vi "7SegmentMod3.vi"() -> ()   [LabVIEW 2014]
doc: "\"Discrete LED demo.vi\" -- Demonstrate a discrete LED connected to a digital output.\n\nInstructions:\n\n-- Click the 'enable blinker' button to toggle between blinking mode\nand static mode.\n-- In static mode, click the 'digital level' button to set the state of the\ndigital output.\n-- The 'digital output state' LED indicator shows the state of the\ndigital output (on = high, off = low)."
uses:
  <vilib>/Utility/error.llb/Error Cluster From Error Code.vi
  <vilib>/myRIO/Common/Instrument Driver Framework/myRIO v1.0/DIO/vis/myRIO v1.0 Write DIO.vi
  <vilib>/myRIO/Instrument Drivers/Onboard IO/DIO/DIO.lvlib
panel:
  in  "Figure-8 Speed":dbl=18.0
  in  "Direction: Figure-8":bool
  in  "Direction: Chase":bool
  in  "Path":enum16{"Chase", "Figure-8"}(ring)
  in  "Chase":dbl=18.0
  out "error out":errorcluster
  in  "error in (no error)":errorcluster
  in  "[ESC]":bool
  # "7-Segment LED demo"
  # "counter-clockwise"
  # "counter-clockwise"
  # "clockwise"
  # "clockwise"
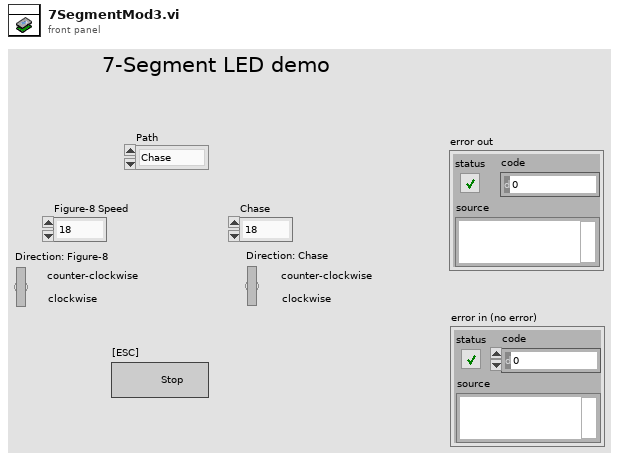
[diagram p1: front panel]
types:
  T1 = typedef "DIO.lvlib/DIO Reference.ctl" = cluster{"myRIO Reference":T2, "DIO Channels List":T6}
  T2 = typedef "myRIO Generic Hardware Reference.ctl" = cluster{"myRIO Model":T3, "myRIO Hardware Reference":T4}
  T3 = typedef "Hardware Version Enum.ctl" = enum16{"Unknown", "myRIO-1900", "myRIO-1950"}
  T4 = typedef "myRIO v1.0 Reference.ctl" = cluster{"Generic FPGA Reference":T5, "Allow multiple opens":bool}
  T5 = typedef "Generic FPGA Reference.ctl" = refnum<k20>
  T6 = typedef "DIO Channels List.ctl" = T7[]
  T7 = typedef "DIO Channels Enum.ctl" = enum16{"Not Connected", "C/DIO0", "C/DIO1", "C/DIO2", "C/DIO3", "C/DIO4", "C/DIO5", "C/DIO6", "C/DIO7", "A/DIO0", "A/DIO1", "A/DIO2", "A/DIO3", "A/DIO4", "A/DIO5", "A/DIO6", "A/DIO7", "A/DIO8", "A/DIO9", "A/DIO10", "A/DIO11", "A/DIO12", "A/DIO13", "A/DIO14", "A/DIO15", "B/DIO0", "B/DIO1", "B/DIO2", "B/DIO3", "B/DIO4", "B/DIO5", "B/DIO6", "B/DIO7", "B/DIO8", "B/DIO9", "B/DIO10", "B/DIO11", "B/DIO12", "B/DIO13", "B/DIO14", "B/DIO15", "LED0", "LED1", "LED2", "LED3", "Button0"}
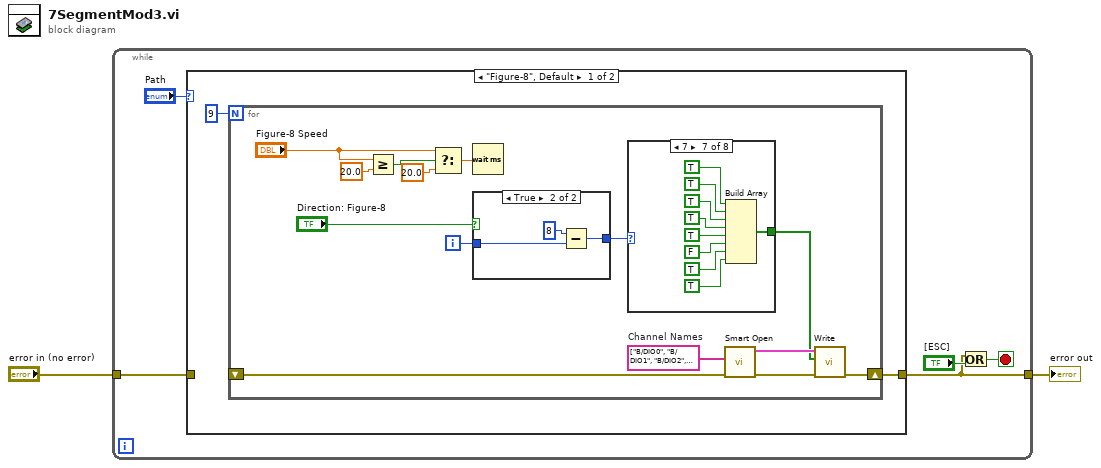
[diagram p0: block diagram]
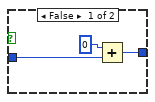
[diagram p2: hidden frame]
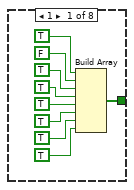
[diagram p3: hidden frame]
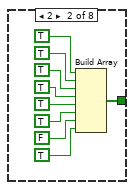
[diagram p4: hidden frame]
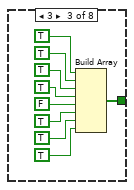
[diagram p5: hidden frame]
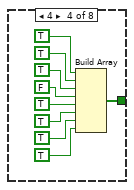
[diagram p6: hidden frame]
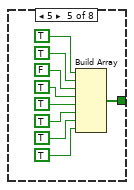
[diagram p7: hidden frame]
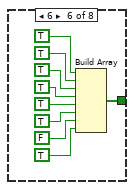
[diagram p8: hidden frame]
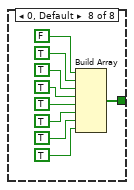
[diagram p9: hidden frame]
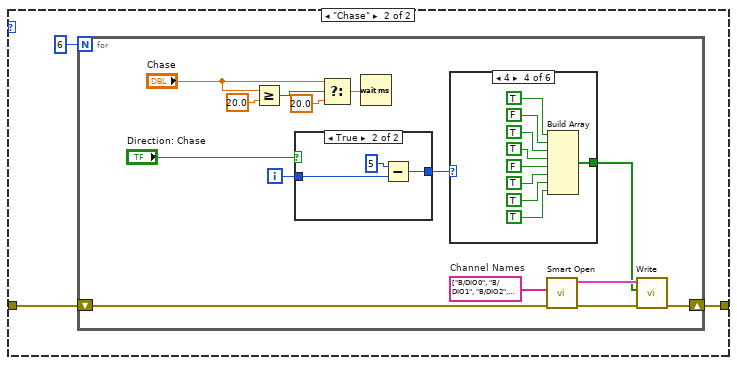
[diagram p10: hidden frame]
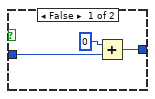
[diagram p11: hidden frame]
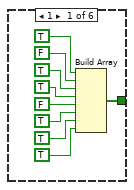
[diagram p12: hidden frame]
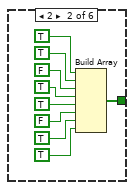
[diagram p13: hidden frame]
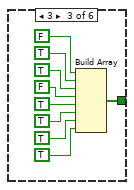
[diagram p14: hidden frame]
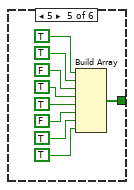
[diagram p15: hidden frame]
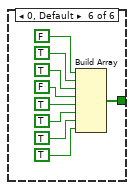
[diagram p16: hidden frame]
diagram:
  n1 = while {
    tunnel: [w5] -> w2
    tunnel: "error in (no error)" -> [w4]
    stop <- w7 stop-if-true
    n2 = case shown="\"Figure-8\", Default" "Path" {
      tunnel: [w8 w104] -> w5
      tunnel: w4 -> [_ w103]
      frame "Figure-8", Default {
        n3 = for {
          N: 9 -> [_]
          shift-right: [w22] -> w8
          shift-left: _ -> [w21]
          i -> [w12]
          w23 = tag[] ["B/DIO0", "B/DIO1", "B/DIO2", "B/DIO3", "B/DIO4", "B/DIO5", "B/DIO6", "B/DIO7"]  # Channel Names
          n4 = Greater Or Equal?(x="Figure-8 Speed", y=20.0) -> (x >= y?=w18:bool)
          n5 = Select(t="Figure-8 Speed", s=w18, f=20.0) -> (s? t:f=w16:dbl)
          n6 = Wait (ms)(milliseconds to wait=w16) -> ()  [unwired: 1 out]
          n7 = case shown="True" "Direction: Figure-8" {
            tunnel: [w25 w28] -> w11
            tunnel: w12 -> [w24 w27]
            frame False {
              n8 = Add(x=0, y=w24) -> (x+y=w25:i32)
            }
            frame True {
              n9 = Subtract(x=8, y=w27) -> (x-y=w28:i32)
            }
          }
          n10 = case shown="7" w11 {
            tunnel: [w30 w39 w48 w57 w66 w75 w84 w93] -> w13
            frame 1 {
              n11 = Build Array(TRUE, FALSE, TRUE, TRUE, TRUE, TRUE, TRUE, TRUE) -> (w30:bool[])
            }
            frame 2 {
              n12 = Build Array(TRUE, TRUE, TRUE, TRUE, TRUE, TRUE, FALSE, TRUE) -> (w39:bool[])
            }
            frame 3 {
              n13 = Build Array(TRUE, TRUE, TRUE, TRUE, FALSE, TRUE, TRUE, TRUE) -> (w48:bool[])
            }
            frame 4 {
              n14 = Build Array(TRUE, TRUE, TRUE, FALSE, TRUE, TRUE, TRUE, TRUE) -> (w57:bool[])
            }
            frame 5 {
              n15 = Build Array(TRUE, TRUE, FALSE, TRUE, TRUE, TRUE, TRUE, TRUE) -> (w66:bool[])
            }
            frame 6 {
              n16 = Build Array(TRUE, TRUE, TRUE, TRUE, TRUE, TRUE, FALSE, TRUE) -> (w75:bool[])
            }
            frame 7 {
              n17 = Build Array(TRUE, TRUE, TRUE, TRUE, TRUE, FALSE, TRUE, TRUE) -> (w84:bool[])
            }
            frame 0, Default {
              n18 = Build Array(FALSE, TRUE, TRUE, TRUE, TRUE, TRUE, TRUE, TRUE) -> (w93:bool[])
            }
          }
          n19 = call <vilib>:"Smart Open.vi"("error in (no error)"=w21, "Channel Names"=w23) -> ("error out"=w14:errorcluster, "DIO Ref Out"=w15:T1)  [unwired: 8 in]
          n20 = call <vilib>:"Write.vi"("error in (no error)"=w14, "Values"=w13, "DIO Ref In"=w15) -> ("error out"=w22:errorcluster)  [unwired: 6 in, 1 out]
        }
      }
      frame "Chase" {
        n21 = for {
          N: 6 -> [_]
          shift-right: [w117] -> w104
          shift-left: w103 -> [w116]
          i -> [w107]
          w118 = tag[] ["B/DIO0", "B/DIO1", "B/DIO2", "B/DIO3", "B/DIO4", "B/DIO5", "B/DIO6", "B/DIO7"]  # Channel Names
          n22 = Greater Or Equal?(x="Chase", y=20.0) -> (x >= y?=w113:bool)
          n23 = case shown="True" "Direction: Chase" {
            tunnel: [w120 w123] -> w106
            tunnel: w107 -> [w119 w122]
            frame False {
              n24 = Add(x=0, y=w119) -> (x+y=w120:i32)
            }
            frame True {
              n25 = Subtract(x=5, y=w122) -> (x-y=w123:i32)
            }
          }
          n26 = Select(t="Chase", s=w113, f=20.0) -> (s? t:f=w111:dbl)
          n27 = Wait (ms)(milliseconds to wait=w111) -> ()  [unwired: 1 out]
          n28 = case shown="4" w106 {
            tunnel: [w125 w134 w143 w152 w161 w170] -> w108
            frame 1 {
              n29 = Build Array(TRUE, FALSE, TRUE, TRUE, FALSE, TRUE, TRUE, TRUE) -> (w125:bool[])
            }
            frame 2 {
              n30 = Build Array(TRUE, TRUE, FALSE, TRUE, TRUE, FALSE, TRUE, TRUE) -> (w134:bool[])
            }
            frame 3 {
              n31 = Build Array(FALSE, TRUE, TRUE, FALSE, TRUE, TRUE, TRUE, TRUE) -> (w143:bool[])
            }
            frame 4 {
              n32 = Build Array(TRUE, FALSE, TRUE, TRUE, FALSE, TRUE, TRUE, TRUE) -> (w152:bool[])
            }
            frame 5 {
              n33 = Build Array(TRUE, TRUE, FALSE, TRUE, TRUE, FALSE, TRUE, TRUE) -> (w161:bool[])
            }
            frame 0, Default {
              n34 = Build Array(FALSE, TRUE, TRUE, FALSE, TRUE, TRUE, TRUE, TRUE) -> (w170:bool[])
            }
          }
          n35 = call <vilib>:"Smart Open.vi"("error in (no error)"=w116, "Channel Names"=w118) -> ("error out"=w109:errorcluster, "DIO Ref Out"=w110:T1)  [unwired: 8 in]
          n36 = call <vilib>:"Write.vi"("error in (no error)"=w109, "Values"=w108, "DIO Ref In"=w110) -> ("error out"=w117:errorcluster)  [unwired: 6 in, 1 out]
        }
      }
    }
    n37 = Or(x=w5, y="[ESC]") -> (x .or. y?=w7:bool)
  }
  "error out" <- w2
